vi "Convert Lines To Polar.vi"(8 "Lines In":T1(array[cluster]) {"End Point"."Y" format="%.2f"; "End Point"."X" format="%.2f"; "Start Point"."Y" format="%.2f"; "Start Point"."X" format="%.2f"}, 10 "Angle In":dbl[](array[numeric]), 11 "Range In":dbl[](array[numeric])) -> (2 "Angle Out":dbl[](array[numeric]), 3 "Range Out":dbl[](array[numeric]))   [LabVIEW 2012]
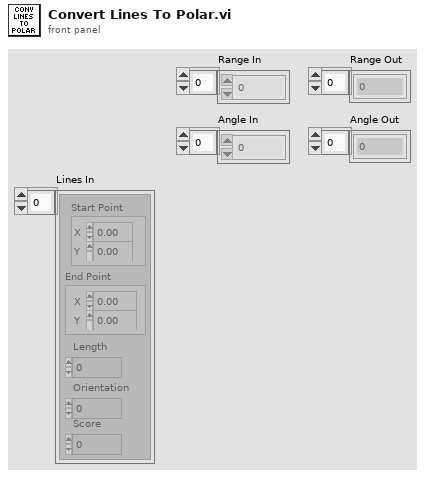
[diagram p1: front panel]
types:
  T1 = cluster{"Start Point":cluster{"X":sgl, "Y":sgl}, "End Point":cluster{"X":sgl, "Y":sgl}, "Length":dbl, "Orientation":dbl, "Score":dbl}[]
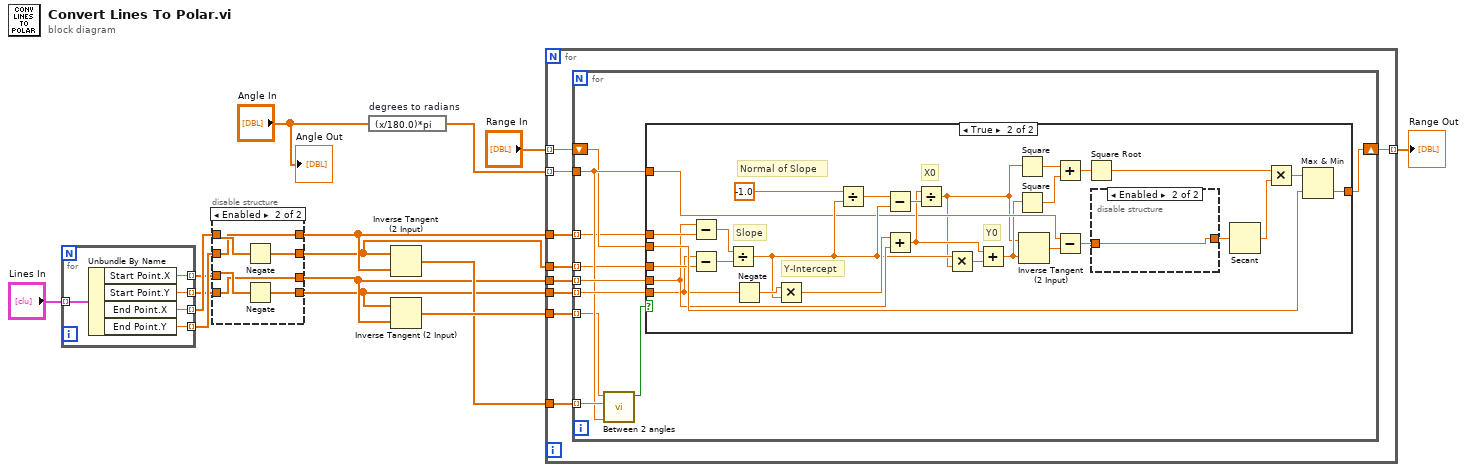
[diagram p0: block diagram]
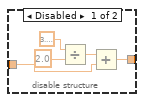
[diagram p4: hidden frame]
diagram:
  n1 = for {
    tunnel: "Lines In" -> [w20] mode=indexing
    tunnel: [w19] -> w5 mode=indexing
    tunnel: [w18] -> w6 mode=indexing
    tunnel: [w17] -> w7 mode=indexing
    tunnel: [w16] -> w8 mode=indexing
    n2 = Unbundle By Name(w20) -> ("Start Point.X"=w19:sgl, "Start Point.Y"=w18:sgl, "End Point.X"=w17:sgl, "End Point.Y"=w16:sgl)
  }
  n3 = disable-structure shown="Enabled" {
    disable-tunnel: [w24 w26] -> w1
    disable-tunnel: w8 -> [w24 w25]
    disable-tunnel: w7 -> [w23 w27]
    disable-tunnel: [w23 w25] -> w2
    disable-tunnel: w6 -> [w22 w28]
    disable-tunnel: [w22 w29] -> w3
    disable-tunnel: [w21 w28] -> w4
    disable-tunnel: w5 -> [w21 w30]
    frame Disabled {
    }
    frame Enabled {
      n4 = Negate(x=w27) -> (-x=w26:sgl[])
      n5 = Negate(x=w30) -> (-x=w29:sgl[])
    }
  }
  n6 = expression code="(x/180.0)*pi" "degrees to radians"("Angle In") -> (w14:dbl[])
  n7 = Inverse Tangent (2 Input)(1:w2, 2:w1) -> (0:w11:sgl[])
  n8 = Inverse Tangent (2 Input)(1:w4, 2:w3) -> (0:w12:sgl[])
  n9 = for {
    tunnel: w14 -> [w37] mode=indexing
    tunnel: "Range In" -> [w36] mode=indexing
    tunnel: w12 -> [w39]
    tunnel: w11 -> [w38]
    tunnel: [w35] -> w10 mode=indexing
    tunnel: w4 -> [w34]
    tunnel: w3 -> [w33]
    tunnel: w1 -> [w32]
    tunnel: w2 -> [w31]
    n10 = for {
      tunnel: w39 -> [w43] mode=indexing
      tunnel: w38 -> [w49] mode=indexing
      tunnel: w37 -> [w44]
      shift-right: [w47] -> w35
      shift-left: w36 -> [w42]
      tunnel: w34 -> [w46] mode=indexing
      tunnel: w33 -> [w45] mode=indexing
      tunnel: w32 -> [w41] mode=indexing
      tunnel: w31 -> [w40] mode=indexing
      n11 = call "Between 2 angles.vi"("Test Angle"=w44, "Angle 2"=w49, "Angle 1"=w43) -> ("Is between Angle 1 and Angle 2"=w48:bool)  [unwired: 8 in]
      n12 = case shown="True" w48 {
        tunnel: [w50 w78] -> w47
        tunnel: w42 -> [w50 w77]
        tunnel: w46 -> [_ w65]
        tunnel: w45 -> [_ w64]
        tunnel: w44 -> [_ w55]
        tunnel: w41 -> [_ w71]
        tunnel: w40 -> [_ w70]
        frame False {
        }
        frame True {
          # "Y0"
          # "X0"
          # "Y-Intercept"
          # "Normal of Slope"
          # "Slope"
          n13 = Subtract(x=w65, y=w70) -> (x-y=w69:sgl)
          n14 = Subtract(x=w64, y=w71) -> (x-y=w68:sgl)
          n15 = Divide(x=w69, y=w68) -> (x/y=w59:sgl)
          n16 = Negate(x=w64) -> (-x=w63:sgl)
          n17 = Multiply(x=w63, y=w59) -> (x*y=w66:sgl)
          n18 = Divide(x=sgl -1.0, y=w59) -> (x/y=w62:sgl)
          n19 = Subtract(x=w62, y=w59) -> (x-y=w61:sgl)
          n20 = Add(x=w66, y=w65) -> (x+y=w57:sgl)
          n21 = Divide(x=w57, y=w61) -> (x/y=w51:sgl)
          n22 = Multiply(x=w59, y=w51) -> (x*y=w58:sgl)
          n23 = Add(x=w57, y=w58) -> (x+y=w52:sgl)
          n24 = Square(x=w51) -> (x^2=w75:sgl)
          n25 = Square(x=w52) -> (x^2=w76:sgl)
          n26 = Inverse Tangent (2 Input)(1:w52, 2:w51) -> (0:w60:sgl)
          n27 = Add(x=w75, y=w76) -> (x+y=w74:sgl)
          n28 = Subtract(x=w55, y=w60) -> (x-y=w53:dbl)
          n29 = Square Root(x=w74) -> (sqrt(x)=w73:sgl)
          n30 = disable-structure shown="Enabled" {
            disable-tunnel: [w80 w84] -> w54
            disable-tunnel: w53 -> [w79 w84]
            frame Disabled {
              n31 = Divide(x=3.141592653589793, y=2.0) -> (x/y=w83:dbl)
              n32 = Add(x=w83, y=w79) -> (x+y=w80:dbl)
            }
            frame Enabled {
            }
          }
          n33 = Secant(1:w54) -> (0:w56:dbl)
          n34 = Multiply(x=w73, y=w56) -> (x*y=w72:dbl)
          n35 = Max & Min(x=w72, y=w77) -> (min(x,y)=w78:dbl)  [unwired: 1 out]
        }
      }
    }
  }
  "Range Out" <- w10
  "Angle Out" <- "Angle In"
